vi "DSF.Engine.Transceiver Thread.Shutdown.vi"(8 "error in (no error)":errorcluster, 11 "Transceiver Thread in":refnum<class "DSF.Engine.Transceiver Thread.lvclass">) -> (0 "error out":errorcluster, 3 "Transceiver Thread out":refnum<class "DSF.Engine.Transceiver Thread.lvclass">)   [LabVIEW 2017, in "DSF.Engine.lvlib" / "DSF.Engine.Transceiver Thread.lvclass"]
uses:
  DSF.Engine.Transceiver Thread.lvclass
  DSF.Engine.Transceiver Thread.lvclass/DSF.Engine.Transceiver Thread.ctl
  DSF.Engine.Transceiver.lvclass
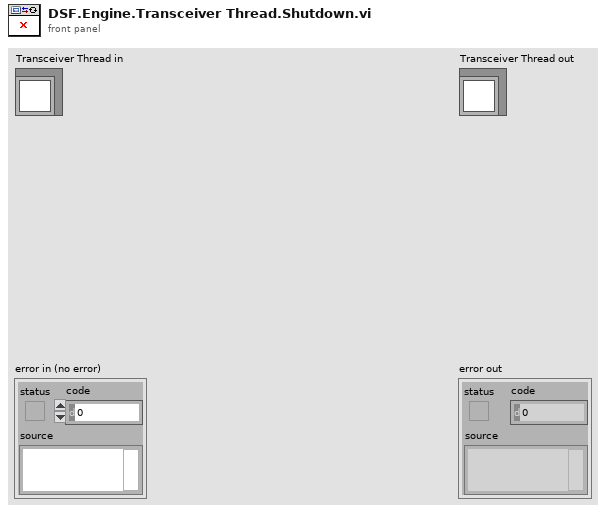
[diagram p1: front panel]
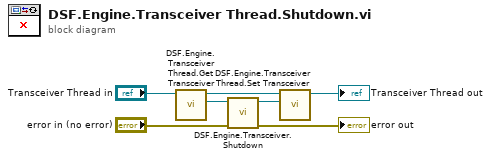
[diagram p0: block diagram]
diagram:
  n1 = call "DSF.Engine.Transceiver Thread.Get Transceiver.vi"("Transceiver Thread in"="Transceiver Thread in") -> ("Transceiver"=w7:refnum<class "DSF.Engine.Transceiver.lvclass">, "Transceiver Thread out"=w5:refnum<class "DSF.Engine.Transceiver Thread.lvclass">)  [unwired: 9 in]
  n2 = call-dynamic "DSF.Engine.Transceiver.Shutdown.vi"("error in (no error)"="error in (no error)", "Transceiver in"=w7) -> ("error out"=→"error out":errorcluster, "Transceiver out"=w6:refnum<class "DSF.Engine.Transceiver.lvclass">)  [unwired: 8 in]
  n3 = call "DSF.Engine.Transceiver Thread.Set Transceiver.vi"("Transceiver"=w6, "Transceiver Thread in"=w5) -> ("Transceiver Thread out"=→"Transceiver Thread out":refnum<class "DSF.Engine.Transceiver Thread.lvclass">)  [unwired: 9 in]
